vi "VIP_Pre-Uninstall Custom Action.vi"(10 "Variant":variant) -> (0 "error out":errorcluster)   [LabVIEW 2021]
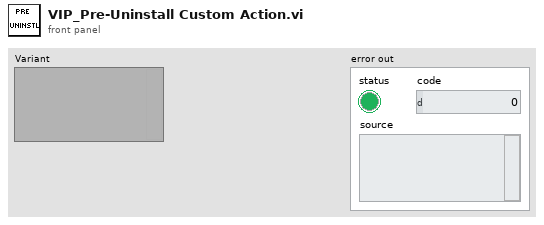
[diagram p1: front panel]
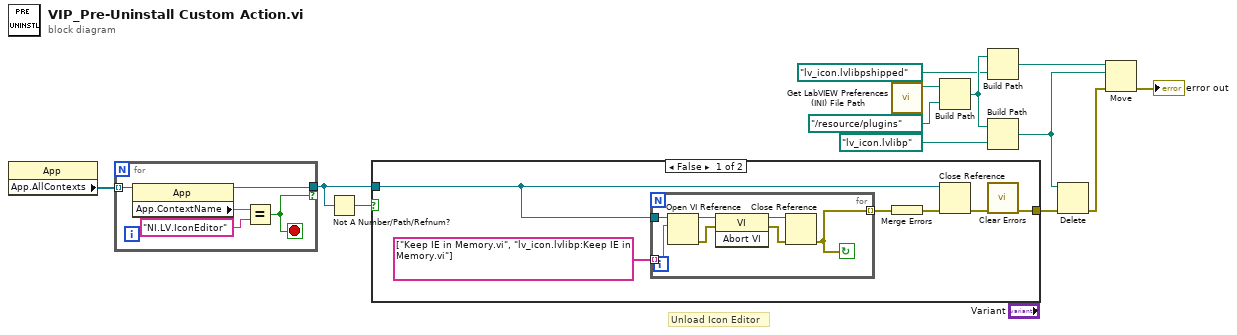
[diagram p0: block diagram]
diagram:
  # "Unload Icon Editor"
  n1 = property class="App"() -> ("App.AllContexts"=w3:refnum<vi>[])  [unwired: 2 in, 2 out]
  n2 = for {
    tunnel: w3 -> [w18] mode=indexing
    tunnel: [w17] -> w2 if=w15
    stop <- w15 stop-if-true
    n3 = property class="App"(reference=w18) -> (reference out=w17:refnum<vi>, "App.ContextName"=w14:string)  [unwired: 1 in, 1 out]
    n4 = Equal?(x=w14, y="NI.LV.IconEditor") -> (x = y?=w15:bool)
  }
  n5 = Not A Number/Path/Refnum?(number/path/refnum=w2) -> (NaN/Path/Refnum?=w1:bool)
  n6 = case shown="False" w1 {
    tunnel: w2 -> [w19 _]
    tunnel: [w22 _] -> w11
    frame False {
      n7 = for {
        tunnel: w19 -> [w27]
        tunnel: string[] ["Keep IE in Memory.vi", "lv_icon.lvlibp:Keep IE in Memory.vi"] -> [w25] mode=indexing
        tunnel: [w29] -> w21 mode=indexing
        stop <- w29 continue-if-true
        n8 = Open VI Reference(application reference (local)=w27, vi path=w25) -> (vi reference=w28:refnum<vi>, error out=w30:errorcluster)  [unwired: 1 in, 3 out]
        n9 = invoke class="VI" method="Abort VI"(reference=w28, error in=w30) -> (reference out=w26:refnum<vi>, error out=w31:errorcluster)  [unwired: 1 in, 1 out]
        n10 = Close Reference(reference=w26, error in (no error)=w31) -> (error out=w29:errorcluster)
      }
      n11 = Merge Errors(w21) -> (w24:errorcluster)
      n12 = Close Reference(reference=w19, error in (no error)=w24) -> (error out=w23:errorcluster)
      n13 = call <vilib>:"Clear Errors.vi"("error in (no error)"=w23) -> ("error out"=w22:errorcluster)  [unwired: 5 in, 1 out]
    }
    frame True {
    }
  }
  n14 = call <resource>:"Get LabVIEW Preferences (INI) File Path.vi"() -> ("LabVIEW Preferences (INI) File Path"=w7:path)  [unwired: 11 in]
  n15 = Build Path(base path=w7, name or relative path=path "../resource/plugins" ("symbolic path")) -> (appended path=w10:path)
  n16 = Build Path(base path=w10, name or relative path=path "lv_icon.lvlibpshipped") -> (appended path=w5:path)
  n17 = Build Path(base path=w10, name or relative path=path "lv_icon.lvlibp") -> (appended path=w4:path)
  n18 = Delete(path (use dialog)=w4, error in=w11) -> (error out=w13:errorcluster)  [unwired: 3 in, 2 out]
  n19 = Move(source path=w5, error in=w13, 10:w4) -> (error out=→"error out":errorcluster)  [unwired: 2 in, 2 out]
